vi "SeCrTs-Data transfer_C.vi"(0 "Data FIFO Ref":T1, 2 "Message Queue":refnum<queue>, 3 "error constant":errorcluster) -> (10 "error out":errorcluster)   [LabVIEW 2022 SP3]
uses:
  RT Controls/SeCrTs-Data FIFO.ctl
  <vilib>/Platform/TimedLoop/XDataNode/timing_clust.ctl
  <vilib>/Platform/TimedLoop/XDataNode/nitl_modes.ctl
  <vilib>/Platform/TimedLoop/XDataNode/wakeup.ctl
  RT Controls/SeCrTs-Data Type Control screen.ctl
  RT Support/SeCrTs-RT_Global_R.vi
  <vilib>/platform/TimedLoop/XDataNode/XDataNode.xnode
  <vilib>/ErrorRing/Error Ring.xnode
  <vilib>/Platform/TimedLoop/XDataNode/XDNodeRunTimeDep.lvlib
  <resource>/objmgr/ni.dex.rc
panel:
  out "Write Backlog":i32
  out "Loop Delay":u32
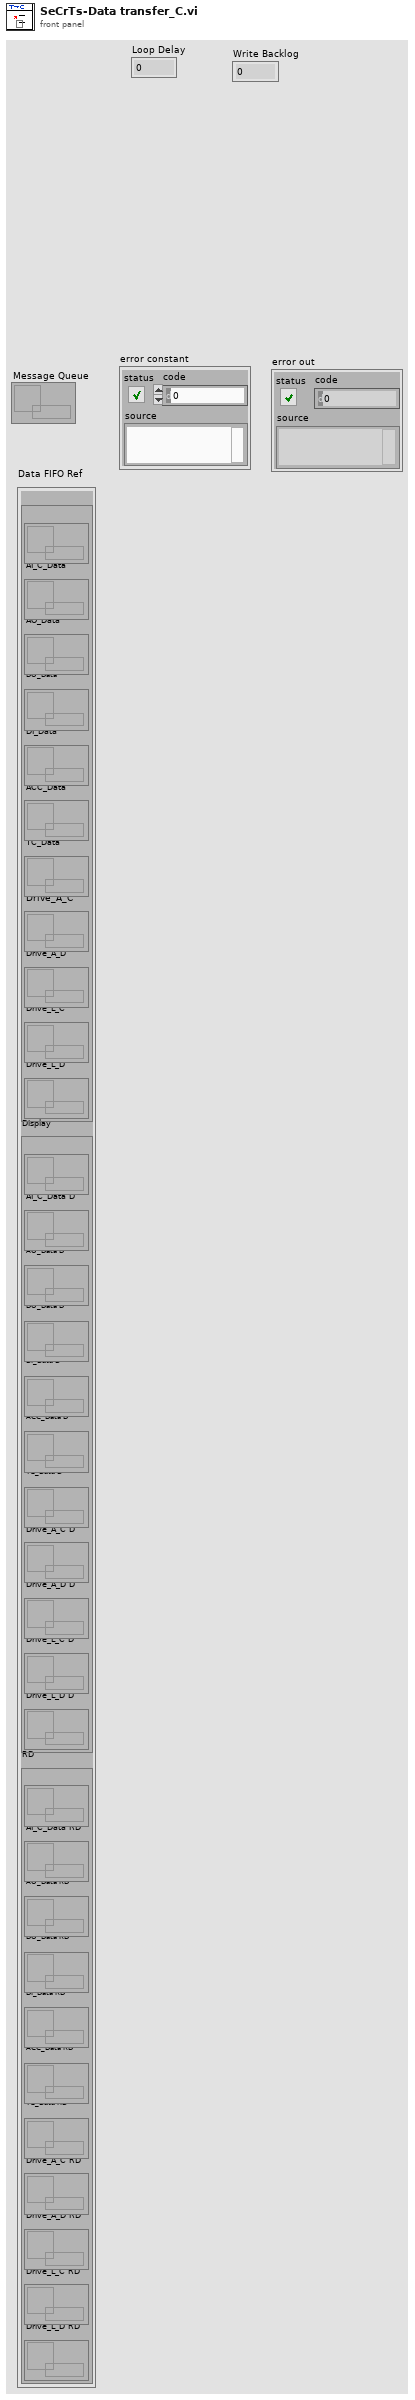
[diagram p1: front panel]
types:
  T1 = typedef "SeCrTs-Data FIFO.ctl" = cluster{"Control":cluster{"AI_V_Data":refnum<queue>, "AI_C_Data":refnum<queue>, "AO_Data":refnum<queue>, "DO_Data":refnum<queue>, "DI_Data":refnum<queue>, "ACC_Data":refnum<queue>, "TC_Data":refnum<queue>, "Drive_A_C":refnum<queue>, "Drive_A_D":refnum<queue>, "Drive_L_C":refnum<queue>, "Drive_L_D":refnum<queue>}, "Display":cluster{"AI_V_Data D":refnum<queue>, "AI_C_Data D":refnum<queue>, "AO_Data D":refnum<queue>, "DO_Data D":refnum<queue>, "DI_Data D":refnum<queue>, "ACC_Data D":refnum<queue>, "TC_Data D":refnum<queue>, "Drive_A_C D":refnum<queue>, "Drive_A_D D":refnum<queue>, "Drive_L_C D":refnum<queue>, "Drive_L_D D":refnum<queue>}, "RD":cluster{"AI_V_Data RD":refnum<queue>, "AI_C_Data RD":refnum<queue>, "AO_Data RD":refnum<queue>, "DO_Data RD":refnum<queue>, "DI_Data RD":refnum<queue>, "ACC_Data RD":refnum<queue>, "TC_Data RD":refnum<queue>, "Drive_A_C RD":refnum<queue>, "Drive_A_D RD":refnum<queue>, "Drive_L_C RD":refnum<queue>, "Drive_L_D RD":refnum<queue>}}
  T2 = typedef "SeCrTs-Data Type Control screen.ctl" = cluster{"DI_Data":digitalwaveform[], "Drive_A_C":waveform(dbl)[], "Drive_A_D":waveform(dbl)[], "Drive_L_C":waveform(dbl)[], "Drive_L_D":waveform(dbl)[], "Loop Status":bool[], "CDT Timer":dbl, "RT Error":cluster{"Error Code":string, "Error Source":string}, "DO":waveform(dbl)[], "SEQ Monitor":string[]}
  T3 = enum16{"Init", "Read 'All'", "Read 'n'", "Read '1'", "Write '1'", "Write 'n'", "Write 'All'"}
  T4 = typedef "XDNodeRunTimeDep.lvlib/timing_clust.ctl" = cluster{"Expected End [f-1]":u64, "Actual End [f-1]":u64, "Finished Late? [f-1]":bool, "Expected End [i-1]":u64, "Actual End [i-1]":u64, "Finished Late? [i-1]":bool, "Expected Start [i]":u64, "Actual Start [i]":u64, "Expected Start [f]":u64, "Actual Start [f]":u64, "Source Name":string, "Structure Name":string, "Period":i64, "Deadline":i64, "Offset":i64, "Start":i64, "Priority":i32, "Timeout":i32, "Mode":T5, "Wakeup Reason":T6, "Error":errorcluster, "Source Type":string, "Secondary Source Type":string, "Global End Time":u64, "Global Start Time":u64, "Frame Duration":u64, "Iteration Duration":u64, "Assigned CPU":i32, "I/O Scan Engine Mode":u32}
  T5 = typedef "XDNodeRunTimeDep.lvlib/nitl_modes.ctl" = enum32{"No Change", "Process missed periods, maintain original phase", "Discard missed periods, maintain original phase", "Process missed periods, ignore original phase", "Discard missed periods, ignore original phase"}
  T6 = typedef "XDNodeRunTimeDep.lvlib/wakeup.ctl" = enum32{"Normal", "Aborted", "Asynchronous wakeup", "Timing source error", "Timed loop error", "Timeout"}
  T7 = cluster{"Start DAQ":bool, "Stop DAQ":bool, "RT Stop":bool, "RT Exit":bool, "Start Seq":bool}
  T8 = cluster{"Error Code":string, "Error Source":string}
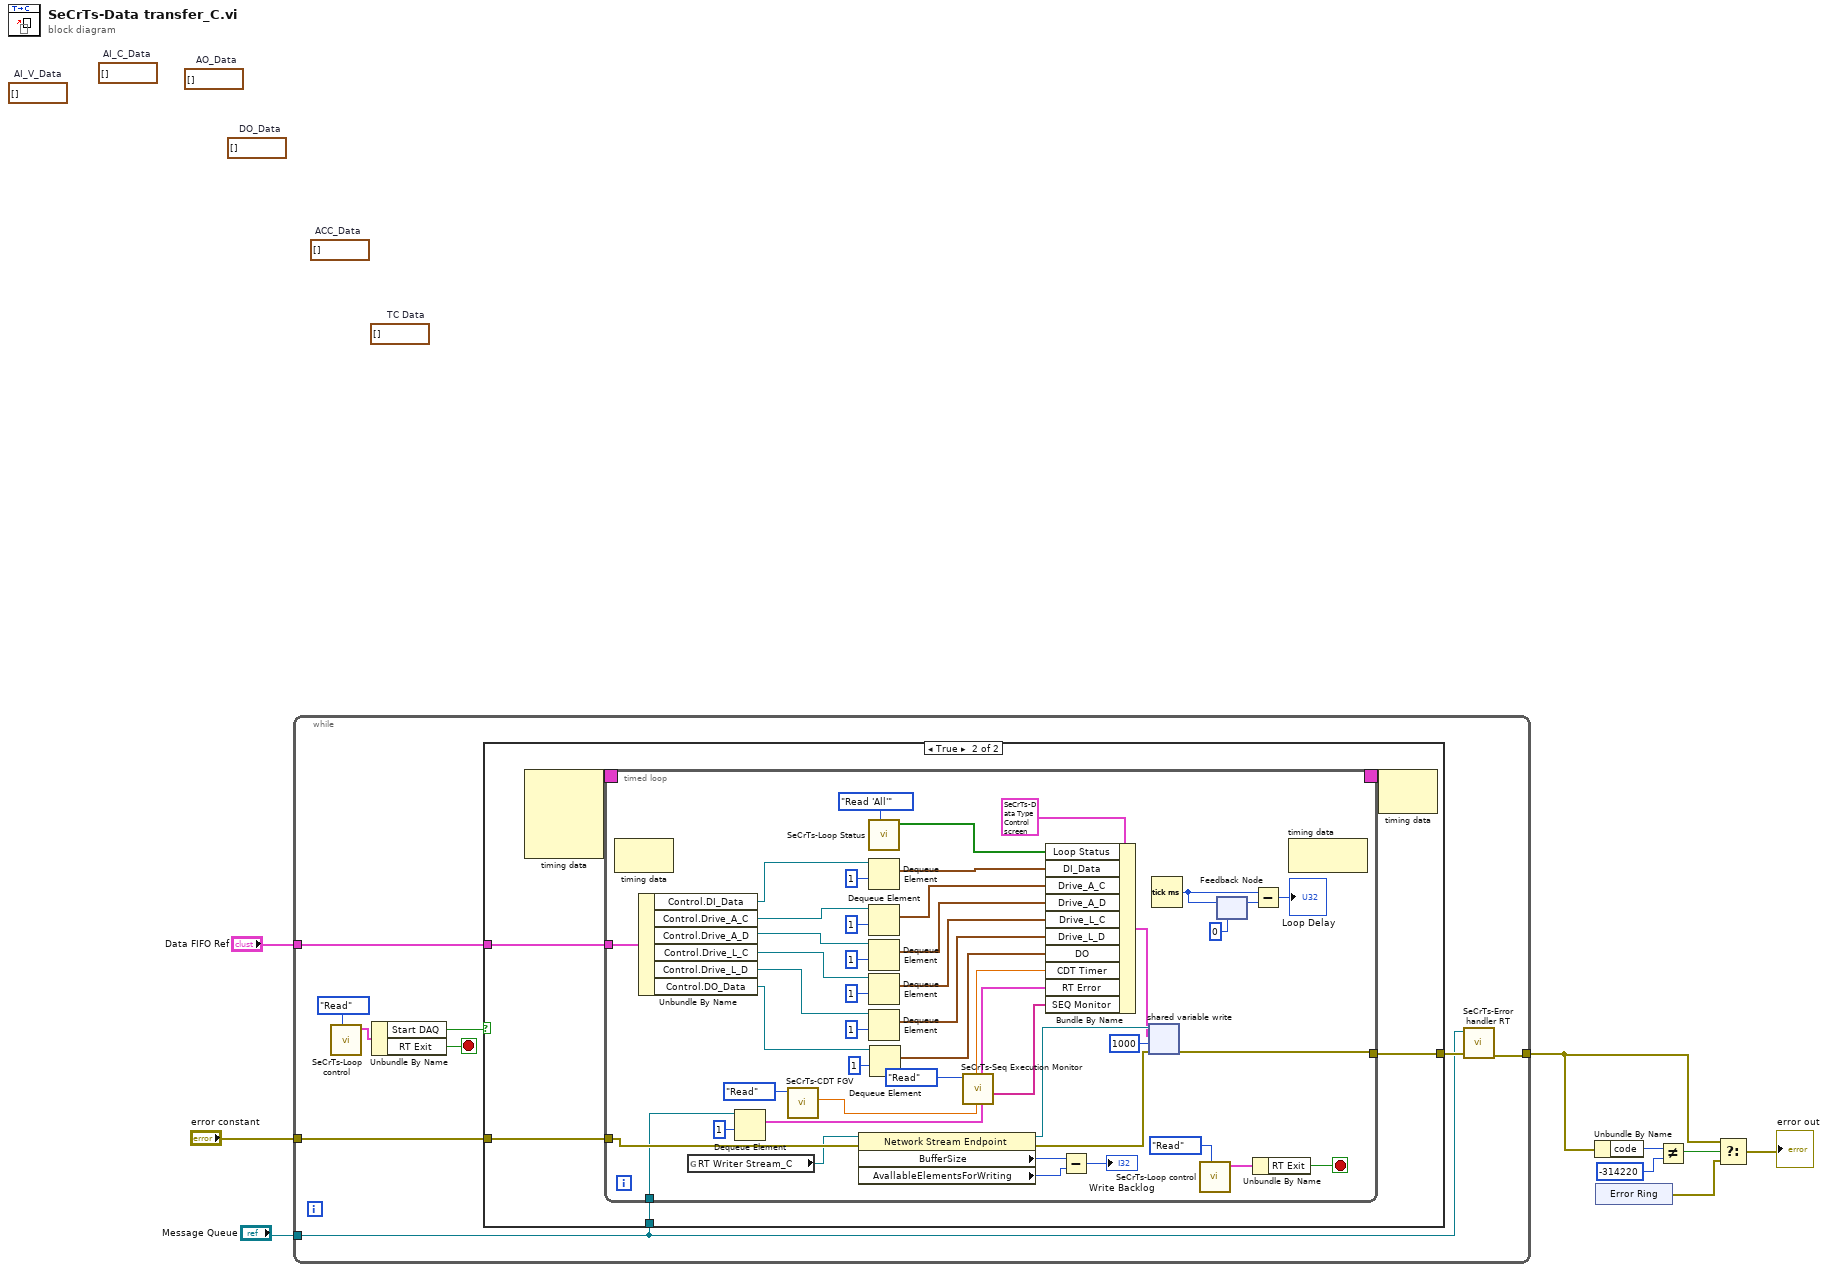
[diagram p0: block diagram]
diagram:
  (unwired) waveform(dbl)[] []  # TC Data
  (unwired) waveform(dbl)[] []  # ACC_Data
  (unwired) waveform(dbl)[] []  # DO_Data
  (unwired) waveform(dbl)[] []  # AO_Data
  (unwired) waveform(dbl)[] []  # AI_C_Data
  (unwired) waveform(dbl)[] []  # AI_V_Data
  n1 = while {
    tunnel: "error constant" -> [w18]
    tunnel: [w11] -> w4
    tunnel: "Data FIFO Ref" -> [w17]
    tunnel: "Message Queue" -> [w10]
    stop <- w13 stop-if-true
    n2 = call "SeCrTs-Loop control.vi"("Action"=enum16{"Init", "Write", "Read"}."Read") -> ("Loop Control out"=w16:T7)  [unwired: 9 in, 1 out]
    n3 = Unbundle By Name(w16) -> ("Start DAQ"=w14:bool, "RT Exit"=w13:bool)
    n4 = case shown="True" w14 {
      tunnel: w18 -> [w19 w25]
      tunnel: [w19 w24] -> w12
      tunnel: w17 -> [_ w21]
      tunnel: w10 -> [_ w20]
      frame False {
      }
      frame True {
        n5 = node-c288() -> (w23:T4)  [unwired: 4 in]
        n6 = timed-loop {
          tunnel: w25 -> [w65]
          tunnel: [w64] -> w24
          timing: w23 -> [_]
          timing-out: [_] -> w22
          tunnel: w21 -> [w59]
          tunnel: w20 -> [w34]
          stop <- w45 stop-if-true
          n7 = node-c288() -> ()  [unwired: 1 in, 1 out]
          n8 = Unbundle By Name(w59) -> ("Control.DI_Data"=w58:refnum<queue>, "Control.Drive_A_C"=w57:refnum<queue>, "Control.Drive_A_D"=w56:refnum<queue>, "Control.Drive_L_C"=w55:refnum<queue>, "Control.Drive_L_D"=w54:refnum<queue>, "Control.DO_Data"=w31:refnum<queue>)
          n9 = global read "SeCrTs-RT_Global_R.vi" "RT Writer Stream_C"() -> (w48:refnum<k21>)
          n10 = Dequeue Element(queue=w34, timeout in ms (-1)=1) -> (element=w28:T8)  [unwired: 1 in, 3 out]
          n11 = call "SeCrTs-CDT FGV.vi"("Write/Read"=enum16{"Write", "Read"}."Read") -> ("CDT Out"=w29:dbl)  [unwired: 9 in, 1 out]
          n12 = property class="Network Stream Endpoint"(reference=w48, error in=w65) -> (reference out=w70:refnum<k21>, error out=w66:errorcluster, "BufferSize"=w69:i32, "AvallableElementsForWriting"=w68:i32)
          n13 = call "SeCrTs-Loop Status.vi"("Option"=T3."Read 'All'") -> ("Status List Out"=w43:bool[])  [unwired: 8 in, 2 out]
          n14 = Dequeue Element(queue=w58, timeout in ms (-1)=1) -> (element=w53:digitalwaveform[])  [unwired: 1 in, 3 out]
          n15 = Dequeue Element(queue=w57, timeout in ms (-1)=1) -> (element=w52:waveform(dbl)[])  [unwired: 1 in, 3 out]
          n16 = Dequeue Element(queue=w56, timeout in ms (-1)=1) -> (element=w51:waveform(dbl)[])  [unwired: 1 in, 3 out]
          n17 = Dequeue Element(queue=w55, timeout in ms (-1)=1) -> (element=w50:waveform(dbl)[])  [unwired: 1 in, 3 out]
          n18 = Dequeue Element(queue=w54, timeout in ms (-1)=1) -> (element=w49:waveform(dbl)[])  [unwired: 1 in, 3 out]
          n19 = Dequeue Element(queue=w31, timeout in ms (-1)=1) -> (element=w30:waveform(dbl)[])  [unwired: 1 in, 3 out]
          n20 = call "SeCrTs-Seq Execution Monitor.vi"("Enum"=enum16{"Read", "Write "}."Read") -> ("Seq Monitor"=w26:string[])  [unwired: 9 in, 1 out]
          n21 = Bundle By Name(cluster=T2 {"DI_Data"=[], "Drive_A_C"=[], "Drive_A_D"=[], "Drive_L_C"=[], "Drive_L_D"=[], "Loop Status"=[], "CDT Timer"=0.0, "RT Error"={"Error Code"="", "Error Source"=""}, "DO"=[], "SEQ Monitor"=[]} ("Cluster"), "Loop Status"=w43, "DI_Data"=w53, "Drive_A_C"=w52, "Drive_A_D"=w51, "Drive_L_C"=w50, "Drive_L_D"=w49, "DO"=w30, "CDT Timer"=w29, "RT Error"=w28, "SEQ Monitor"=w26) -> (w41:T2)
          n22 = Subtract(x=w69, y=w68) -> (x-y=→"Write Backlog":i32)
          n23 = shared-variable-write(w70, w66, w41, 1000 ("timeout ms (-1)")) -> (w64:errorcluster)  [unwired: 2 out]
          n24 = Tick Count (ms)() -> (millisecond timer value=w61:u32)
          n25 = call "SeCrTs-Loop control.vi"("Action"=enum16{"Init", "Write", "Read"}."Read") -> ("Loop Control out"=w47:T7)  [unwired: 9 in, 1 out]
          n26 = feedback #1(u32 0 ("millisecond timer value")) -> (w62:u32)
          n27 = feedback-in #1(w61) -> ()
          n28 = Subtract(x=w61, y=w62) -> (x-y=→"Loop Delay":u32)
          n29 = Unbundle By Name(w47) -> ("RT Exit"=w45:bool)
          n30 = node-c288() -> ()  [unwired: 1 in, 1 out]
        }
        n31 = node-c288(w22) -> ()  [unwired: 1 out]
      }
    }
    n32 = call "SeCrTs-Error handler RT.vi"("error in"=w12, "Message Queue"=w10) -> ("error out"=w11:errorcluster)  [unwired: 8 in, 1 out]
  }
  n33 = Unbundle By Name(w4) -> ("code"=w9:i32)
  n34 = xnode "Error Ring"() -> ("error out"=w5:errorcluster)
  n35 = Not Equal?(x=w9, y=-314220) -> (x != y?=w6:bool)
  n36 = Select(t=w4, s=w6, f=w5) -> (s? t:f=→"error out":errorcluster)
